vi "Config_ReadFile.vi"(0 "Section":T5(ring), 5 "Config file name":path=path "C:/Users/ceslab/Documents/CES LabView/Configuration/CES_Config_test.ini", 11 "error in":errorcluster) -> (3 "BBB config data":T3, 4 "Actions data":string[][](array[string]), 6 "State data":string[][](array[string]), 8 "Calculation config data":T1, 10 "state_elements":T4, 14 "Spectrometer config data":T2, 15 "error out":errorcluster)   [LabVIEW 2025]
uses:
  BBB/TypeDef_Network.ctl
  TypeDef_SpectrometerConfigData.ctl
  TypeDef_CalculationConfigData.ctl
  <vilib>/Utility/config.llb/Read Key (I32).vi
  <vilib>/Utility/config.llb/Read Key (String).vi
  <vilib>/Utility/config.llb/Read Key (Double).vi
  <vilib>/Utility/config.llb/NI_LVConfig.lvlib
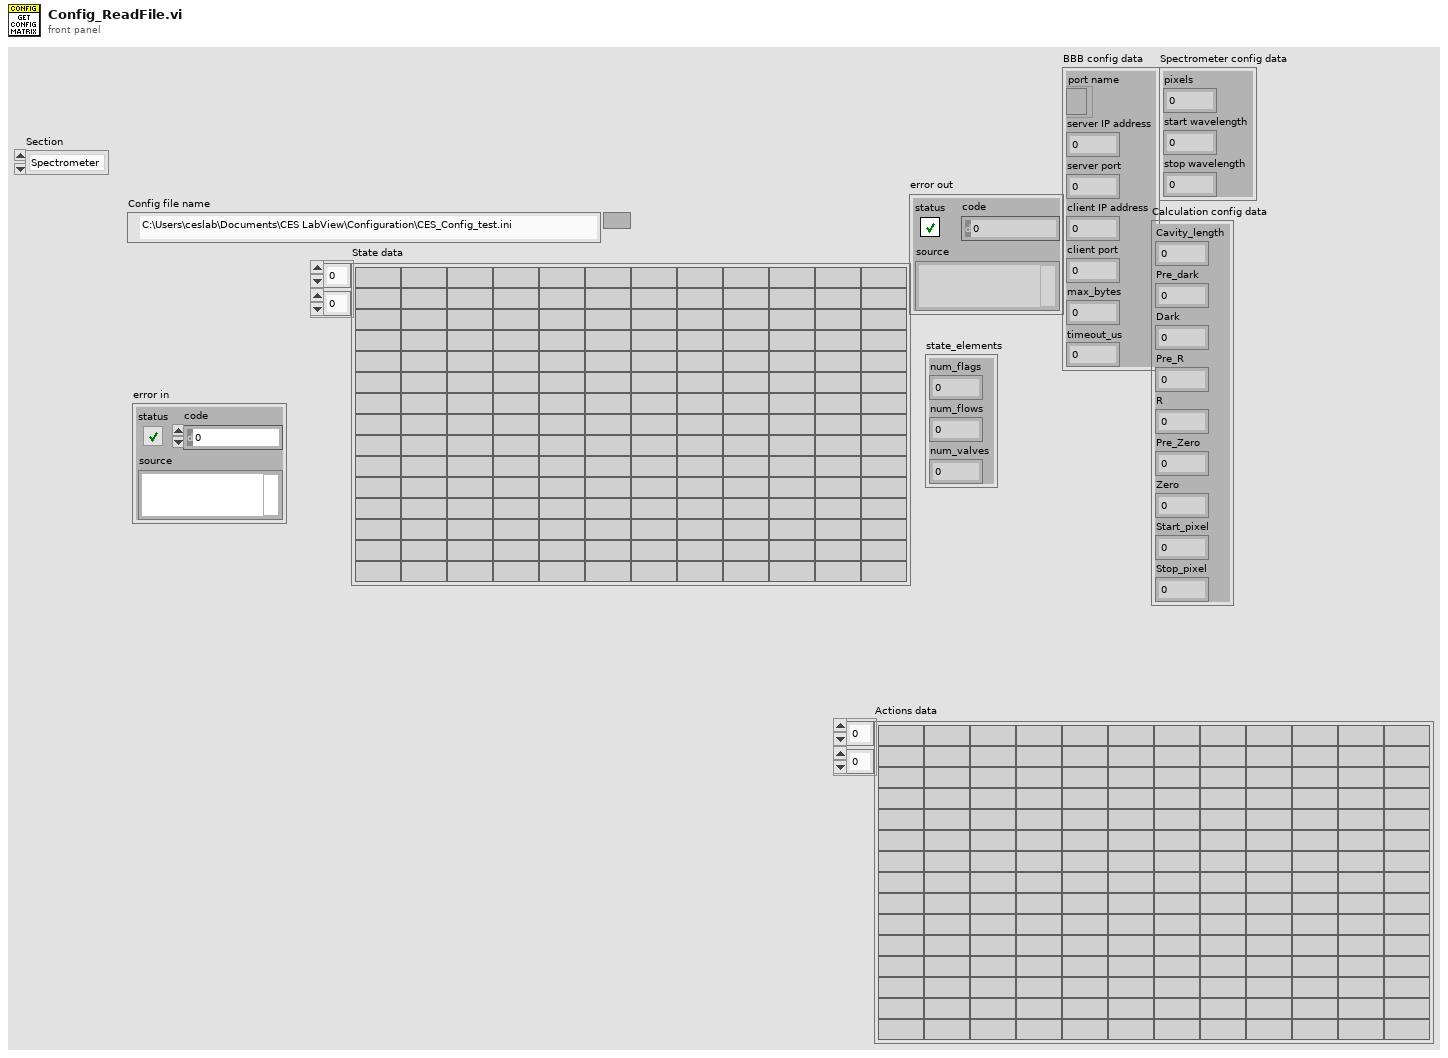
[diagram p1: front panel]
types:
  T1 = typedef "TypeDef_CalculationConfigData.ctl" = cluster{"Cavity_length":dbl, "Pre_dark":i32, "Dark":i32, "Pre_R":i32, "R":i32, "Pre_Zero":i32, "Zero":i32, "Start_pixel":i32, "Stop_pixel":i32}
  T2 = typedef "TypeDef_SpectrometerConfigData.ctl" = cluster{"pixels":i32, "start wavelength":dbl, "stop wavelength":dbl}
  T3 = typedef "TypeDef_Network.ctl" = cluster{"port name":refnum<k16>, "server IP address":u32, "server port":u16, "client IP address":u32, "client port":u16, "max_bytes":i32, "timeout_us":i32}
  T4 = cluster{"num_flags":i32, "num_flows":i32, "num_valves":i32}
  T5 = enum16{"Spectrometer", "Calculations", "BBB", "States", "Actions"}
  T6 = typedef "NI_LVConfig.lvlib/Config Data RefNum.ctl" = refnum<k1>
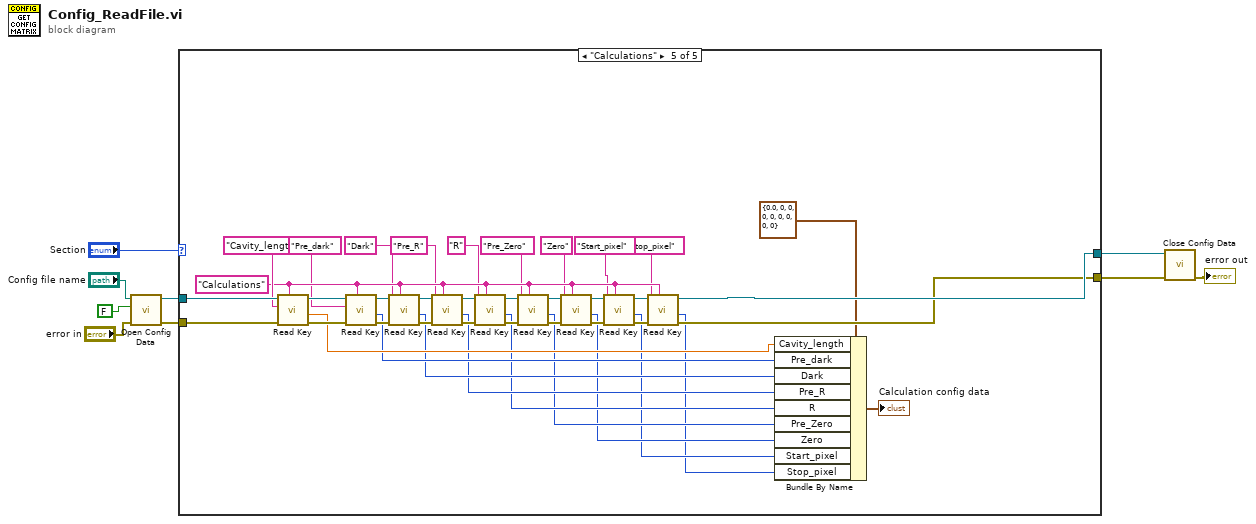
[diagram p0: block diagram]
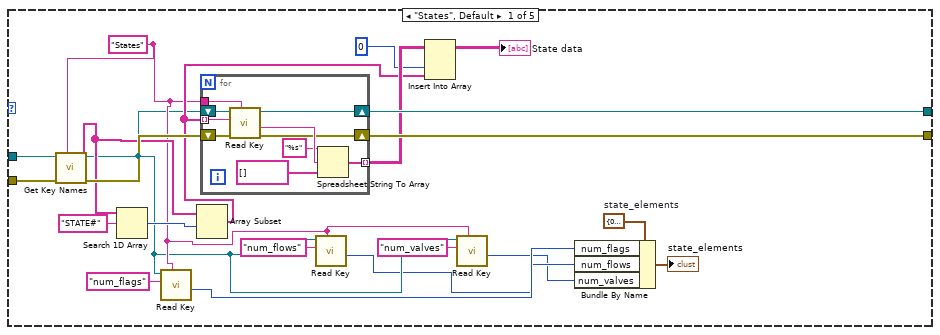
[diagram p2: hidden frame]
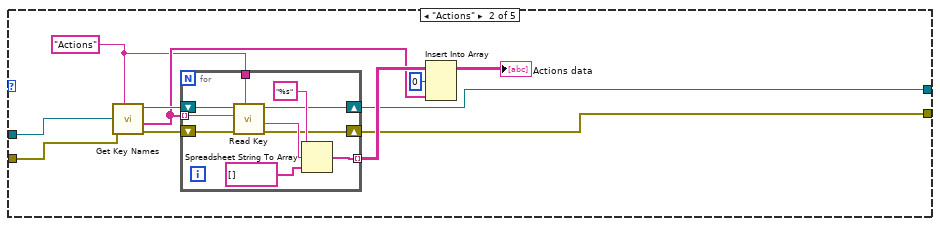
[diagram p3: hidden frame]
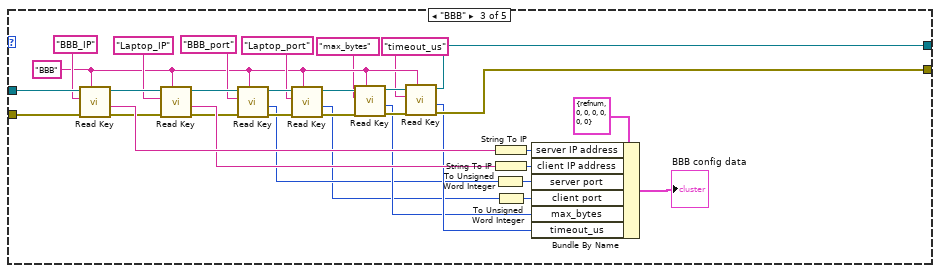
[diagram p4: hidden frame]
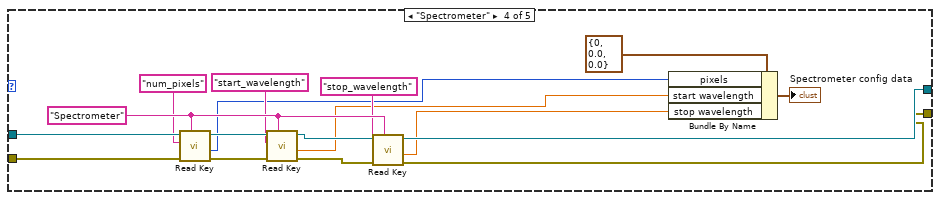
[diagram p5: hidden frame]
diagram:
  n1 = call <vilib>:"Open Config Data.vi"("error in (no error)"="error in", "create file if necessary (T)"=FALSE, "configuration file path"="Config file name") -> ("error out"=w4:errorcluster, "refnum"=w5:T6)  [unwired: 6 in, 1 out]
  n2 = case shown="\"Calculations\"" "Section" {
    tunnel: w5 -> [w28 w46 w95 w112 w153]
    tunnel: w4 -> [w27 w45 w94 w111 w152]
    tunnel: [w30 w42 w77 w107 w127] -> w2
    tunnel: [w29 w43 w74 w105 w126] -> w1
    frame "States", Default {
      w14 = T4 {"num_flags"=0, "num_flows"=0, "num_valves"=0}  # state_elements
      w17 = "States" ("Section")
      n3 = call <vilib>:"Get Key Names.vi"("section"=w17, "error in (no error)"=w27, "refnum"=w28) -> ("error out"=w31:errorcluster, "key names"=w20:string[], "refnum out"=w16:T6)  [unwired: 5 in, 1 out]
      n4 = Search 1D Array(1D array=w20, element="STATE#") -> (index of element=w22:i32)  [unwired: 1 in]
      n5 = call-poly <vilib>:"Read Key.vi"("section"=w17, "key"="num_flags", "refnum"=w16) -> ("value"=w13:i32)  [unwired: 5 in, 3 out]
      n6 = Array Subset(array=w20, index=w22) -> (w21:string[])  [unwired: 1 in]
      n7 = for {
        tunnel: w21 -> [w41] mode=indexing
        tunnel: w17 -> [w40]
        tunnel: [w38] -> w25 mode=indexing
        shift-right: [w33] -> w30
        shift-left: w16 -> [w39]
        shift-right: [w32] -> w29
        shift-left: w31 -> [w34]
        n8 = call-poly <vilib>:"Read Key.vi"("section"=w40, "error in (no error)"=w34, "key"=w41, "refnum"=w39) -> ("error out"=w32:errorcluster, "value"=w36:string, "refnum out"=w33:T6)  [unwired: 4 in, 1 out]
        n9 = Spreadsheet String To Array(format string="%s" ("spreadsheet string"), spreadsheet string=w36, array type (2D Dbl)=string[] []) -> (array=w38:string[])  [unwired: 1 in]
      }
      n10 = call-poly <vilib>:"Read Key.vi"("section"=w17, "key"="num_flows", "refnum"=w16) -> ("value"=w12:i32)  [unwired: 5 in, 3 out]
      n11 = Insert Into Array(array=w25, index (col)=0 ("disabled index (col)"), new element=w21) -> (→"State data":string[][])  [unwired: 1 in]
      n12 = call-poly <vilib>:"Read Key.vi"("section"=w17, "key"="num_valves", "refnum"=w16) -> ("value"=w11:i32)  [unwired: 5 in, 3 out]
      n13 = Bundle By Name(cluster=w14, "num_flags"=w13, "num_flows"=w12, "num_valves"=w11) -> (→"state_elements":T4)
    }
    frame "Actions" {
      w44 = "Actions"
      n14 = call <vilib>:"Get Key Names.vi"("section"=w44, "error in (no error)"=w45, "refnum"=w46) -> ("error out"=w51:errorcluster, "key names"=w49:string[], "refnum out"=w52:T6)  [unwired: 5 in, 1 out]
      n15 = for {
        tunnel: w49 -> [w62] mode=indexing
        tunnel: [w60] -> w50 mode=indexing
        shift-right: [w55] -> w42
        shift-left: w52 -> [w61]
        shift-right: [w54] -> w43
        shift-left: w51 -> [w56]
        tunnel: w44 -> [w53]
        n16 = call-poly <vilib>:"Read Key.vi"("section"=w53, "error in (no error)"=w56, "key"=w62, "refnum"=w61) -> ("error out"=w54:errorcluster, "value"=w58:string, "refnum out"=w55:T6)  [unwired: 4 in, 1 out]
        n17 = Spreadsheet String To Array(format string="%s" ("spreadsheet string"), spreadsheet string=w58, array type (2D Dbl)=string[] []) -> (array=w60:string[])  [unwired: 1 in]
      }
      n18 = Insert Into Array(array=w50, index (col)=0 ("disabled index (col)"), new element=w49) -> (→"Actions data":string[][])  [unwired: 1 in]
    }
    frame "BBB" {
      w72 = "BBB" ("section")
      n19 = call-poly <vilib>:"Read Key.vi"("section"=w72, "error in (no error)"=w94, "key"="BBB_IP", "refnum"=w95) -> ("error out"=w82:errorcluster, "value"=w87:string, "refnum out"=w93:T6)  [unwired: 4 in, 1 out]
      n20 = call-poly <vilib>:"Read Key.vi"("section"=w72, "error in (no error)"=w82, "key"="Laptop_IP", "refnum"=w93) -> ("error out"=w81:errorcluster, "value"=w85:string, "refnum out"=w92:T6)  [unwired: 4 in, 1 out]
      n21 = call-poly <vilib>:"Read Key.vi"("section"=w72, "error in (no error)"=w81, "key"="BBB_port", "refnum"=w92) -> ("error out"=w80:errorcluster, "value"=w67:i32, "refnum out"=w83:T6)  [unwired: 4 in, 1 out]
      n22 = call-poly <vilib>:"Read Key.vi"("section"=w72, "error in (no error)"=w80, "key"="Laptop_port", "refnum"=w83) -> ("error out"=w76:errorcluster, "value"=w64:i32, "refnum out"=w79:T6)  [unwired: 4 in, 1 out]
      n23 = call-poly <vilib>:"Read Key.vi"("section"=w72, "error in (no error)"=w76, "key"="max_bytes", "refnum"=w79) -> ("error out"=w75:errorcluster, "value"=w68:i32, "refnum out"=w78:T6)  [unwired: 4 in, 1 out]
      n24 = call-poly <vilib>:"Read Key.vi"("section"=w72, "error in (no error)"=w75, "key"="timeout_us", "refnum"=w78) -> ("error out"=w74:errorcluster, "value"=w69:i32, "refnum out"=w77:T6)  [unwired: 4 in, 1 out]
      n25 = To Unsigned Word Integer(number=w67) -> (unsigned 16bit integer=w65:u16)
      n26 = String To IP(1:w87) -> (0:w86:u32)
      n27 = String To IP(1:w85) -> (0:w66:u32)
      n28 = To Unsigned Word Integer(number=w64) -> (unsigned 16bit integer=w63:u16)
      n29 = Bundle By Name(cluster=T3 {"port name"=refnum, "server IP address"=0, "server port"=0, "client IP address"=0, "client port"=0, "max_bytes"=0, "timeout_us"=0}, "server IP address"=w86, "client IP address"=w66, "server port"=w65, "client port"=w63, "max_bytes"=w68, "timeout_us"=w69) -> (→"BBB config data":T3)
    }
    frame "Spectrometer" {
      w104 = "Spectrometer" ("section")
      n30 = call-poly <vilib>:"Read Key.vi"("section"=w104, "error in (no error)"=w111, "key"="num_pixels", "refnum"=w112) -> ("error out"=w109:errorcluster, "value"=w99:i32, "refnum out"=w110:T6)  [unwired: 4 in, 1 out]
      n31 = call-poly <vilib>:"Read Key.vi"("section"=w104, "error in (no error)"=w109, "key"="start_wavelength", "refnum"=w110) -> ("error out"=w106:errorcluster, "value"=w98:dbl, "refnum out"=w108:T6)  [unwired: 4 in, 1 out]
      n32 = call-poly <vilib>:"Read Key.vi"("section"=w104, "error in (no error)"=w106, "key"="stop_wavelength", "refnum"=w108) -> ("error out"=w105:errorcluster, "value"=w97:dbl, "refnum out"=w107:T6)  [unwired: 4 in, 1 out]
      n33 = Bundle By Name(cluster=T2 {"pixels"=0, "start wavelength"=0.0, "stop wavelength"=0.0}, "pixels"=w99, "start wavelength"=w98, "stop wavelength"=w97) -> (→"Spectrometer config data":T2)
    }
    frame "Calculations" {
      w134 = "Calculations" ("section")
      n34 = call-poly <vilib>:"Read Key.vi"("section"=w134, "error in (no error)"=w152, "key"="Cavity_length", "refnum"=w153) -> ("error out"=w149:errorcluster, "value"=w122:dbl, "refnum out"=w150:T6)  [unwired: 4 in, 1 out]
      n35 = call-poly <vilib>:"Read Key.vi"("section"=w134, "error in (no error)"=w149, "key"="Pre_dark", "refnum"=w150) -> ("error out"=w141:errorcluster, "value"=w121:i32, "refnum out"=w148:T6)  [unwired: 4 in, 1 out]
      n36 = call-poly <vilib>:"Read Key.vi"("section"=w134, "error in (no error)"=w141, "key"="Dark", "refnum"=w148) -> ("error out"=w140:errorcluster, "value"=w120:i32, "refnum out"=w147:T6)  [unwired: 4 in, 1 out]
      n37 = call-poly <vilib>:"Read Key.vi"("section"=w134, "error in (no error)"=w140, "key"="Pre_R", "refnum"=w147) -> ("error out"=w139:errorcluster, "value"=w119:i32, "refnum out"=w146:T6)  [unwired: 4 in, 1 out]
      n38 = call-poly <vilib>:"Read Key.vi"("section"=w134, "error in (no error)"=w139, "key"="R", "refnum"=w146) -> ("error out"=w138:errorcluster, "value"=w118:i32, "refnum out"=w145:T6)  [unwired: 4 in, 1 out]
      n39 = call-poly <vilib>:"Read Key.vi"("section"=w134, "error in (no error)"=w138, "key"="Pre_Zero", "refnum"=w145) -> ("error out"=w137:errorcluster, "value"=w117:i32, "refnum out"=w144:T6)  [unwired: 4 in, 1 out]
      n40 = call-poly <vilib>:"Read Key.vi"("section"=w134, "error in (no error)"=w137, "key"="Zero", "refnum"=w144) -> ("error out"=w136:errorcluster, "value"=w116:i32, "refnum out"=w143:T6)  [unwired: 4 in, 1 out]
      n41 = call-poly <vilib>:"Read Key.vi"("section"=w134, "error in (no error)"=w136, "key"="Start_pixel", "refnum"=w143) -> ("error out"=w135:errorcluster, "value"=w115:i32, "refnum out"=w142:T6)  [unwired: 4 in, 1 out]
      n42 = call-poly <vilib>:"Read Key.vi"("section"=w134, "error in (no error)"=w135, "key"="Stop_pixel", "refnum"=w142) -> ("error out"=w126:errorcluster, "value"=w114:i32, "refnum out"=w127:T6)  [unwired: 4 in, 1 out]
      n43 = Bundle By Name(cluster=T1 {"Cavity_length"=0.0, "Pre_dark"=0, "Dark"=0, "Pre_R"=0, "R"=0, "Pre_Zero"=0, "Zero"=0, "Start_pixel"=0, "Stop_pixel"=0}, "Cavity_length"=w122, "Pre_dark"=w121, "Dark"=w120, "Pre_R"=w119, "R"=w118, "Pre_Zero"=w117, "Zero"=w116, "Start_pixel"=w115, "Stop_pixel"=w114) -> (→"Calculation config data":T1)
    }
  }
  n44 = call <vilib>:"Close Config Data.vi"("error in (no error)"=w1, "refnum"=w2) -> ("error out"=→"error out":errorcluster)  [unwired: 8 in, 1 out]
